vi "Send command.vi"(3 "Value":u16, 4 "Command":T1=17 items=["Measured main TEC temperature"=0, "Measured SHG heater temperature"=1, "Measured BRF heater temperature"=2, "Main TEC temperature command"=3, "SHG heater temperature command"=4, "BRF heater temperature command"=5, "Main TEC drive"=6, "SHG heater drive"=7, "BRF heater drive"=8, "Output power from photodiode"=9, "Output power setpoint (Get)"=10, "Output power setpoint (Set)"=11, "Start-up power setting (Get)"=12, "Start-up power setting (Set)"=13, "Measured LDD current"=14, "Maximum LDD current limit"=15, "16-bit fault code"=16, "Head serial number"=17, "Head board rev"=18, "Head type"=19, "LDD enable state"=20, "Key switch command (Get)"=24, "Key switch command (Set)"=25, "Key switch actual"=26, "Interlock status"=27, "Head hours"=28, "Photo or current mode command (Get)"=29, "Photo or current mode command (Set)"=30, "Photo or current mode actual"=31, "Analog input enable command (Get)"=32, "Analog input enable command (Set)"=33, "Analog input actual"=34, "Power supply glue input"=36, "Power supply glue output"=37], 5 "Device handle":u64) -> (0 "Error":errorcluster, 1 "response value":sgl, 2 "response":string)   [LabVIEW 2018]
uses:
  Commands.ctl
  Coherent global.vi
panel:
  # "PN 06/11/2014\n      08/04/2019"
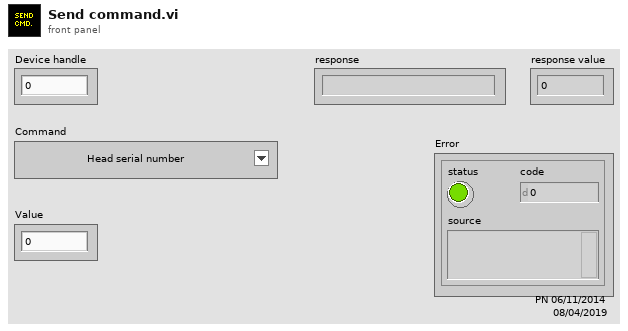
[diagram p1: front panel]
types:
  T1 = typedef "Commands.ctl" = u8
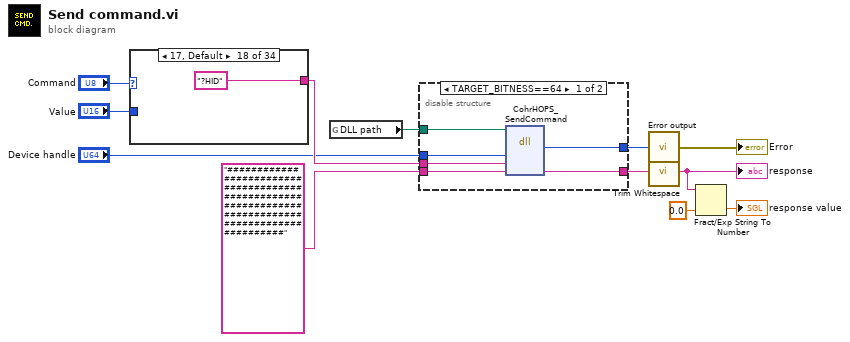
[diagram p0: block diagram]
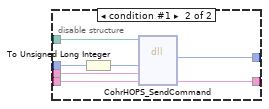
[diagram p2: hidden frame]
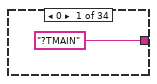
[diagram p3: hidden frame]
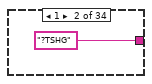
[diagram p4: hidden frame]
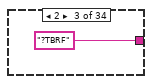
[diagram p5: hidden frame]
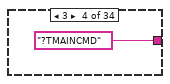
[diagram p6: hidden frame]
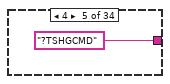
[diagram p7: hidden frame]
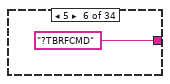
[diagram p8: hidden frame]
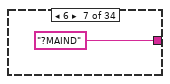
[diagram p9: hidden frame]
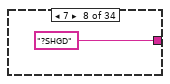
[diagram p10: hidden frame]
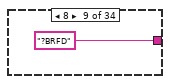
[diagram p11: hidden frame]
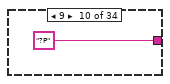
[diagram p12: hidden frame]
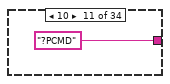
[diagram p13: hidden frame]
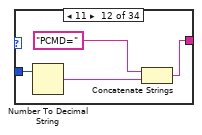
[diagram p14: hidden frame]
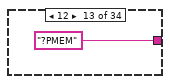
[diagram p15: hidden frame]
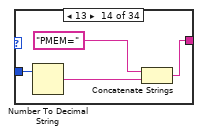
[diagram p16: hidden frame]
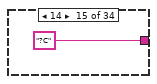
[diagram p17: hidden frame]
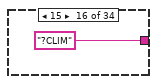
[diagram p18: hidden frame]
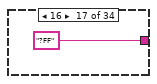
[diagram p19: hidden frame]
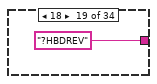
[diagram p20: hidden frame]
diagram:
  n1 = case shown="17, Default" "Command" {
    tunnel: ["?TMAIN" "?TSHG" "?TBRF" "?TMAINCMD" "?TSHGCMD" "?TBRFCMD" "?MAIND" "?SHGD" "?BRFD" "?P" "?PCMD" w24 "?PMEM" w29 "?C" "?CLIM" "?FF" "?HID" "?HBDREV" "?HTYPE" "?L" "?KSWCMD" w42 "?KSW" "?INT" "?HH" "?CMODECMD" w50 "?CMODE" "?ANACMD" w56 "?ANA" "?PSGLUEIN" "?PSGLUEOUT"] -> w10
    tunnel: "Value" -> [_ _ _ _ _ _ _ _ _ _ _ w27 _ w32 _ _ _ _ _ _ _ _ w44 _ _ _ _ w52 _ _ w58 _ _ _]
    frame 0 {
    }
    frame 1 {
    }
    frame 2 {
    }
    frame 3 {
    }
    frame 4 {
    }
    frame 5 {
    }
    frame 6 {
    }
    frame 7 {
    }
    frame 8 {
    }
    frame 9 {
    }
    frame 10 {
    }
    frame 11 {
      n2 = Number To Decimal String(number=w27) -> (decimal integer string=w26:string)  [unwired: 1 in]
      n3 = Concatenate Strings("PCMD=", w26) -> (w24:string)
    }
    frame 12 {
    }
    frame 13 {
      n4 = Number To Decimal String(number=w32) -> (decimal integer string=w31:string)  [unwired: 1 in]
      n5 = Concatenate Strings("PMEM=", w31) -> (w29:string)
    }
    frame 14 {
    }
    frame 15 {
    }
    frame 16 {
    }
    frame 17, Default {
    }
    frame 18 {
    }
    frame 19 {
    }
    frame 20 {
    }
    frame 24 {
    }
    frame 25 {
      n6 = Number To Decimal String(number=w44) -> (decimal integer string=w41:string)  [unwired: 1 in]
      n7 = Concatenate Strings("KSWCMD=", w41) -> (w42:string)
    }
    frame 26 {
    }
    frame 27 {
    }
    frame 28 {
    }
    frame 29 {
    }
    frame 30 {
      n8 = Number To Decimal String(number=w52) -> (decimal integer string=w49:string)  [unwired: 1 in]
      n9 = Concatenate Strings("CMODECMD=", w49) -> (w50:string)
    }
    frame 31 {
    }
    frame 32 {
    }
    frame 33 {
      n10 = Number To Decimal String(number=w58) -> (decimal integer string=w55:string)  [unwired: 1 in]
      n11 = Concatenate Strings("ANACMD=", w55) -> (w56:string)
    }
    frame 34 {
    }
    frame 36 {
    }
    frame 37 {
    }
  }
  n12 = global read "Coherent global.vi" "DLL path"() -> (w1:path)
  n13 = disable-structure shown="TARGET_BITNESS==64" {
    disable-tunnel: "####################################################################################################" ("headType") -> [w67 w71]
    disable-tunnel: w10 -> [w66 w72]
    disable-tunnel: [w65 w69] -> w9
    disable-tunnel: [w64 w70] -> w8
    disable-tunnel: "Device handle" -> [w63 w73]
    disable-tunnel: w1 -> [w62 w74]
    frame condition #0 (active) {
      n14 = dll-call lib="?" fn="CohrHOPS_SendCommand"(path in=w62, "handle"=w63, "command"=w66, "response"=w67) -> ("return value"=w65:i32, "response"=w64:string)  [unwired: 4 in, 2 out]
    }
    frame condition #1 {
      n15 = To Unsigned Long Integer(number=w73) -> (unsigned 32bit integer=w68:u32)
      n16 = dll-call lib="?" fn="CohrHOPS_SendCommand"(path in=w74, "handle"=w68, "command"=w72, "response"=w71) -> ("return value"=w69:i32, "response"=w70:string)  [unwired: 4 in, 2 out]
    }
  }
  n17 = call "Error output.vi"("I32 err code"=w9) -> ("Error Out"=→"Error":errorcluster)
  n18 = call <vilib>:"Trim Whitespace.vi"("string"=w8) -> ("trimmed string"=w4:string)  [unwired: 1 in]
  "response" <- w4
  n19 = Fract/Exp String To Number(string=w4, default (0 dbl)=sgl 0.0 ("default (0 DBL)")) -> (number=→"response value":sgl)  [unwired: 2 in, 1 out]
